vi "DestroyForceDelete.vi"(0 "reference in":refnum<class "G#BaseClass1.lvclass">, 5 "error in (no error)":errorcluster) -> (14 "reference out":refnum<class "G#BaseClass1.lvclass">, 19 "error out":errorcluster)   [LabVIEW 2017, in "G#BaseClass1.lvclass"]
doc: "Destructor."
uses:
  G#BaseClass1.lvclass
  C:/Program Files/National Instruments/LabVIEW 2017/vi.lib/addons/_AddQ/G#Object/G#Object.lvclass
  <vilib>/addons/_AddQ/G#Object/G#Object.lvclass
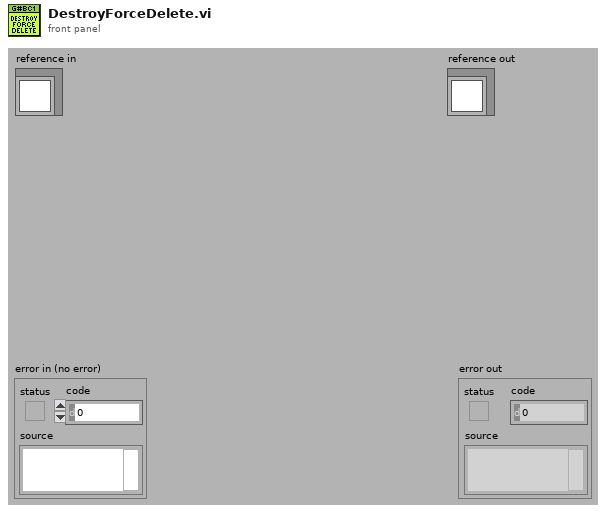
[diagram p1: front panel]
types:
  T1 = typedef "G#BaseClass1.lvclass/ObjectAttributes.ctl" = cluster{"Numeric":dbl, "Array":dbl[]}
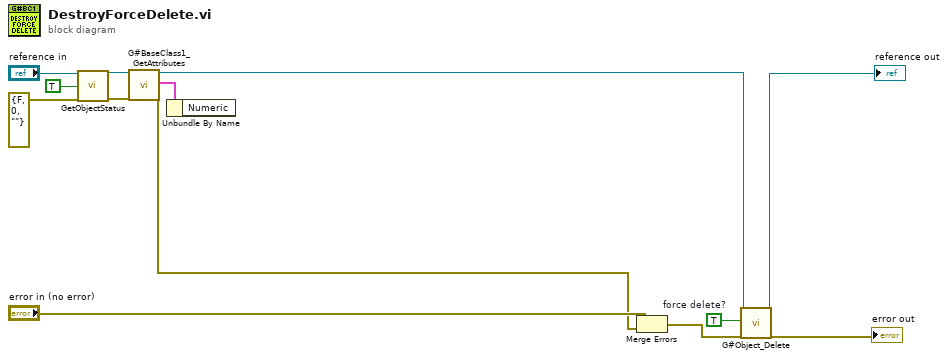
[diagram p0: block diagram]
diagram:
  w1 = TRUE  # force delete?
  n1 = call-dynamic "GetObjectStatus.vi"("reference in"="reference in", "simple info (F)"=TRUE ("simple info"), "error in (no error)"=errorcluster {"status"=FALSE, "code"=0, "source"=""}) -> ("reference out"=w5:refnum<class "G#BaseClass1.lvclass">, "error out"=w6:errorcluster)  [unwired: 5 in, 10 out]
  n2 = call "G#BaseClass1_GetAttributes.vi"("reference in"=w5, "error in (no error)"=w6) -> ("reference out"=w3:refnum<class "G#BaseClass1.lvclass">, "attributes"=w4:T1, "error out"=w7:errorcluster)  [unwired: 14 in, 1 out]
  n3 = Unbundle By Name(w4) -> ()  [unwired: 1 out]
  n4 = Merge Errors("error in (no error)", w7) -> (w2:errorcluster)
  n5 = call <vilib>:"G#Object_Delete.vi"("reference in"=w3, "force delete? (F)"=w1, "error in (no error)"=w2) -> ("reference out"=→"reference out":refnum<class "G#BaseClass1.lvclass">, "error out"=→"error out":errorcluster)  [unwired: 15 in]
